vi "readConfigTel.vi"(8 "error in (no error)":errorcluster, 11 "Path in":T1) -> (0 "error out":errorcluster, 2 "regTel":string[][](array[string]), 3 "Path out":T1)   [LabVIEW 2018]
doc: "Read the telemetry from default.ini file that will be registered by TCP Server.\n\nNOTE: this is only for internal use. User does not call this function directly."
uses:
  <vilib>/Utility/config.llb/Config Data RefNum.ctl
  <vilib>/Utility/config.llb/NI_LVConfig.lvlib
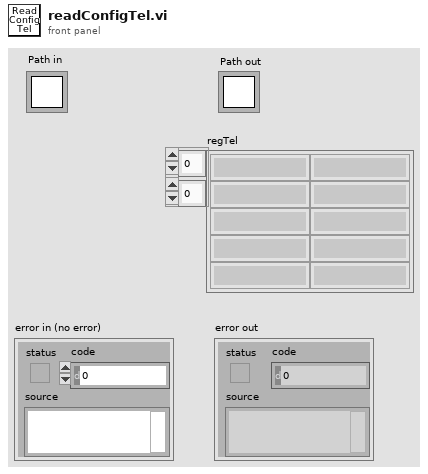
[diagram p1: front panel]
types:
  T1 = typedef "NI_LVConfig.lvlib/Config Data RefNum.ctl" = refnum<k1>
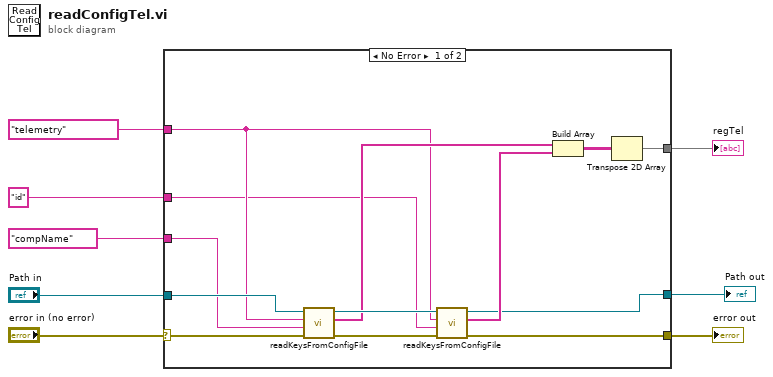
[diagram p0: block diagram]
diagram:
  n1 = case shown="No Error" "error in (no error)" {
    selector: "error in (no error)" -> [w21 w23]
    tunnel: "compName" -> [w10 _]
    tunnel: "telemetry" -> [w11 _]
    tunnel: [w14 w22] -> w3
    tunnel: [w12 w23] -> w5
    tunnel: "Path in" -> [w20 w22]
    tunnel: [w15 _] -> w2
    tunnel: "id" -> [w9 _]
    frame No Error {
      n2 = call "readKeysFromConfigFile.vi"("error in (no error)"=w21, "keys"=w10, "section"=w11, "Refnum in"=w20) -> ("error out"=w13:errorcluster, "arrayOfKeys"=w18:string[], "Refnum out"=w19:T1)  [unwired: 5 in]
      n3 = call "readKeysFromConfigFile.vi"("error in (no error)"=w13, "keys"=w9, "section"=w11, "Refnum in"=w19) -> ("error out"=w12:errorcluster, "arrayOfKeys"=w17:string[], "Refnum out"=w14:T1)  [unwired: 5 in]
      n4 = Build Array(w18, w17) -> (w16:string[][])
      n5 = Transpose 2D Array(2D array=w16) -> (transposed array=w15:string[][])
    }
    frame Error {
    }
  }
  "regTel" <- w2
  "error out" <- w5
  "Path out" <- w3
